vi "TemperatureSensor.vi"() -> (0 "Temperature":dbl)   [LabVIEW 2023]
uses:
  <vilib>/numeric/sub_Random U32.vi
  <vilib>/numeric/Random Number (Range) DBL.vi
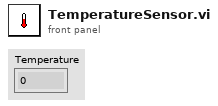
[diagram p1: front panel]
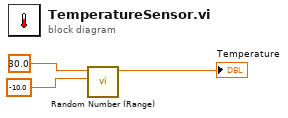
[diagram p0: block diagram]
diagram:
  n1 = call-poly <vilib>:"Random Number (Range).vi"("lower bound (0)"=-10.0, "upper bound (100)"=30.0) -> ("number"=→"Temperature":dbl)  [unwired: 9 in]
